vi "Workshop Exercise 2 Solution.vi"() -> ()   [LabVIEW 2019]
panel:
  out "Table":string[][](table)
  out "Raw Tab-Delimited Data":string
  out "Graph":dbl[][](graph)
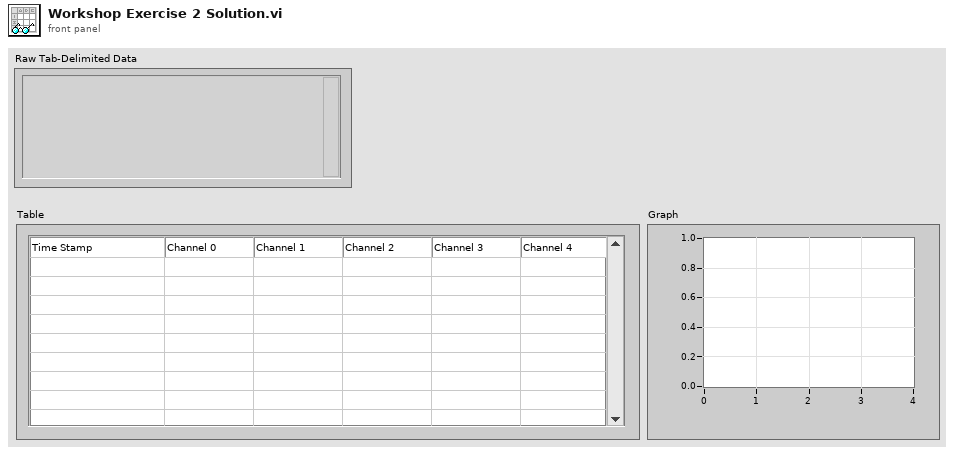
[diagram p1: front panel]
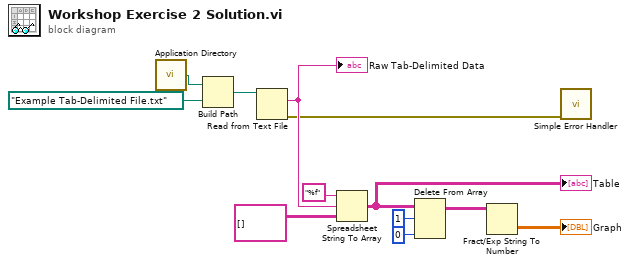
[diagram p0: block diagram]
diagram:
  n1 = call <vilib>:"Application Directory.vi"() -> ("Application Directory"=w2:path)
  n2 = Build Path(base path=w2, name or relative path=path "Example Tab-Delimited File.txt" ("default name")) -> (appended path=w5:path)
  n3 = Read from Text File(file (use dialog)=w5) -> (text=w8:string, error out=w6:errorcluster)  [unwired: 2 in, 3 out]
  "Raw Tab-Delimited Data" <- w8
  n4 = Spreadsheet String To Array(format string="%f", spreadsheet string=w8, array type (2D Dbl)=string[][] [] ("Array")) -> (array=w1:string[][])  [unwired: 1 in]
  "Table" <- w1
  n5 = Delete From Array(array=w1, length=1, index (col)=0 ("disabled index (col)")) -> (array with subset deleted=w3:string[][])  [unwired: 1 in, 1 out]
  n6 = Fract/Exp String To Number(string=w3) -> (number=→"Graph":dbl[][])  [unwired: 4 out]
  n7 = call <vilib>:"Simple Error Handler.vi"("error in (no error)"=w6) -> ()  [unwired: 1 in, 8 out]
